vi "Untitled 2.vi"() -> ()   [LabVIEW 2021]
uses:
  <vilib>/NI/DCAF/Modules/modbus/module channel/Modbus Module Channel.lvclass
panel:
  in  "modbus channels":refnum<class "Modbus Module Channel.lvclass">[](array[class])
  out "error out":errorcluster
  in  "error in":errorcluster
  in  "selected path":path
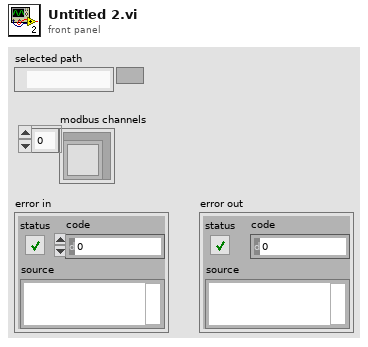
[diagram p1: front panel]
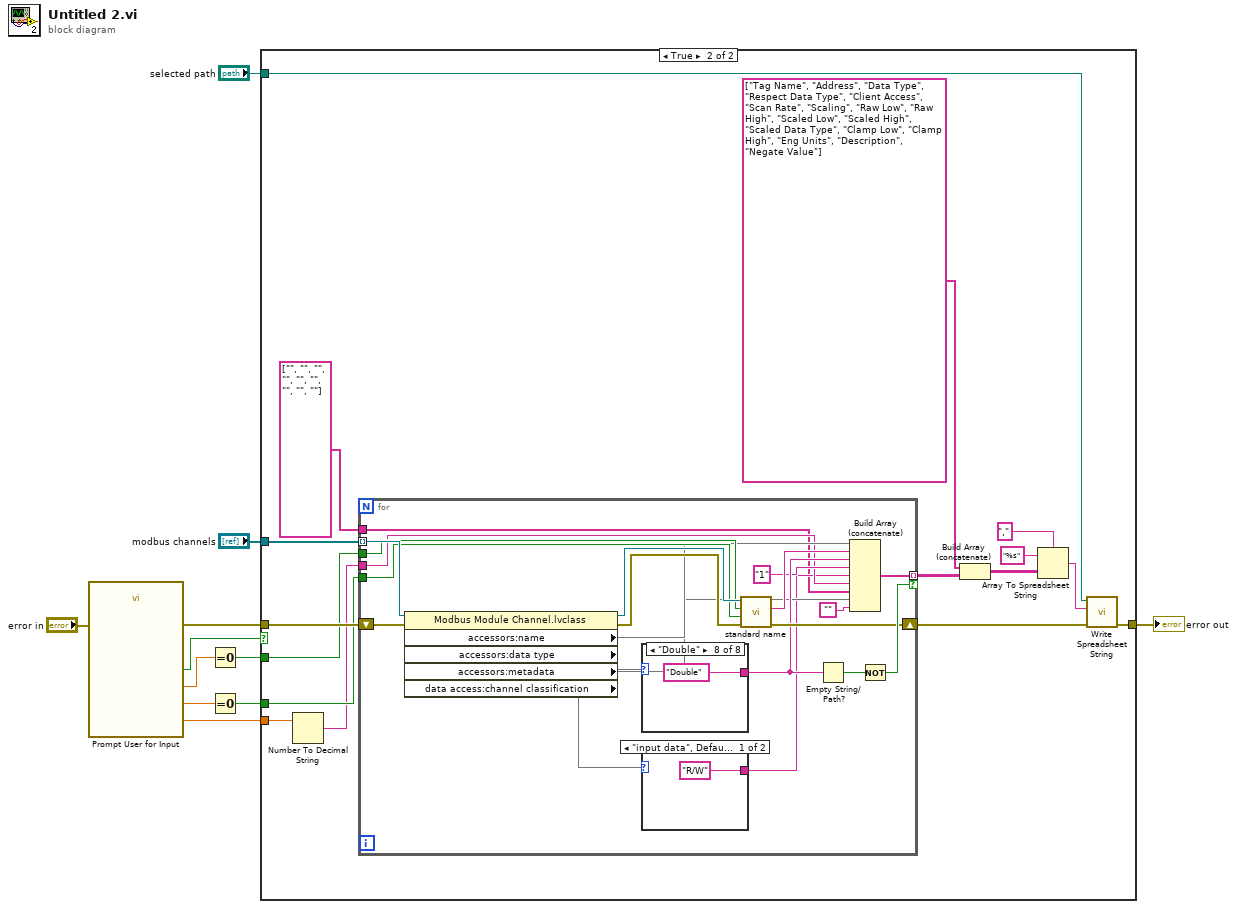
[diagram p0: block diagram]
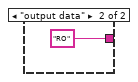
[diagram p3: hidden frame]
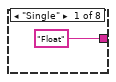
[diagram p4: hidden frame]
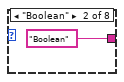
[diagram p5: hidden frame]
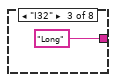
[diagram p6: hidden frame]
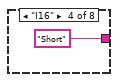
[diagram p7: hidden frame]
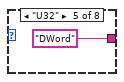
[diagram p8: hidden frame]
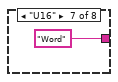
[diagram p10: hidden frame]
diagram:
  n1 = call "Prompt User for Input"("error in (no error)"="error in") -> ("Scan Rate (ms)"=w1:dbl, "Indexing for booleans (0 or 1)"=w5:dbl, "Indexing for register (0 or 1)"=w4:dbl, "OK"=w6:bool, "error out"=w7:errorcluster)  [unwired: 14 in]
  n2 = Equal To 0?(x=w4) -> (x = 0?=w3:bool)
  n3 = Equal To 0?(x=w5) -> (x = 0?=w2:bool)
  n4 = case shown="True" w6 {
    tunnel: "selected path" -> [_ w28]
    tunnel: [w12 w22] -> w10
    tunnel: "modbus channels" -> [_ w21]
    tunnel: w7 -> [w12 w20]
    tunnel: w3 -> [_ w19]
    tunnel: w2 -> [_ w18]
    tunnel: w1 -> [_ w15]
    frame False {
    }
    frame True {
      n5 = Number To Decimal String(number=w15) -> (decimal integer string=w14:string)  [unwired: 1 in]
      n6 = for {
        tunnel: w21 -> [w48] mode=indexing
        shift-right: [w41] -> w23
        shift-left: w20 -> [w49]
        tunnel: [w47] -> w26 mode=indexing if=w45
        tunnel: w19 -> [w40]
        tunnel: w18 -> [w39]
        tunnel: w14 -> [w32]
        tunnel: string[] ["", "", "", "", "", "", "", "", ""] ("array") -> [w29]
        n7 = property class="Modbus Module Channel.lvclass"(reference=w48, error in=w49) -> (reference out=w43:refnum<class "Modbus Module Channel.lvclass">, error out=w42:errorcluster, "accessors:name"=w38, "accessors:data type"=w46, "accessors:metadata"=w34, "data access:channel classification"=w31)
        n8 = case shown="\"Double\"" w46 {
          tunnel: ["Float" "Boolean" "Long" "Short" "DWord" _ "Word" "Double"] -> w36
          frame "Single" {
          }
          frame "Boolean" {
          }
          frame "I32" {
          }
          frame "I16" {
          }
          frame "U32" {
          }
          frame Default {
          }
          frame "U16" {
          }
          frame "Double" {
          }
        }
        n9 = case shown="\"input data\", Default" w31 {
          tunnel: ["R/W" ("element") "RO" ("element")] -> w30
          frame "input data", Default {
          }
          frame "output data" {
          }
        }
        n10 = call <vilib>:"standard name.vi"("error in"=w42, "zero index bit"=w39, "zero index element"=w40, "Modbus Module Channel in"=w43) -> ("error out"=w41:errorcluster, "standard name"=w37:string)  [unwired: 5 in, 1 out]
        n11 = Empty String/Path?(string/path=w36) -> (empty?=w44:bool)
        n12 = Build Array (concatenate)(w38, w37, w36, "1" ("element"), w30, w32, w29, w34, "") -> (w47:string[])
        n13 = Not(x=w44) -> (.not. x?=w45:bool)
      }
      n14 = Build Array (concatenate)(string[] ["Tag Name", "Address", "Data Type", "Respect Data Type", "Client Access", "Scan Rate", "Scaling", "Raw Low", "Raw High", "Scaled Low", "Scaled High", "Scaled Data Type", "Clamp Low", "Clamp High", "Eng Units", "Description", "Negate Value"] ("array"), w26) -> (w17:string[][])
      n15 = Array To Spreadsheet String(delimiter (Tab)="," ("delimiter (\\t)"), array=w17, 3:"%s" ("format (%s)")) -> (spreadsheet string=w24:string)
      n16 = call <vilib>:"Write Spreadsheet String.vi"("error in"=w23, "spreadsheet string"=w24, "file path (dialog if empty)"=w28) -> ("error out"=w22:errorcluster)  [unwired: 7 in, 1 out]
    }
  }
  "error out" <- w10
